vi "Exe_folder_path.vi"(8 "error in (no error)":errorcluster) -> (0 "error out":errorcluster, 2 "One level up":string, 3 "Exe folder":string)   [LabVIEW 2013]
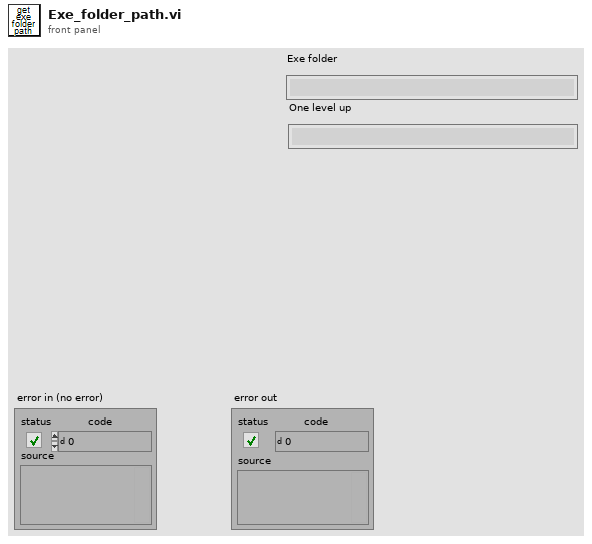
[diagram p1: front panel]
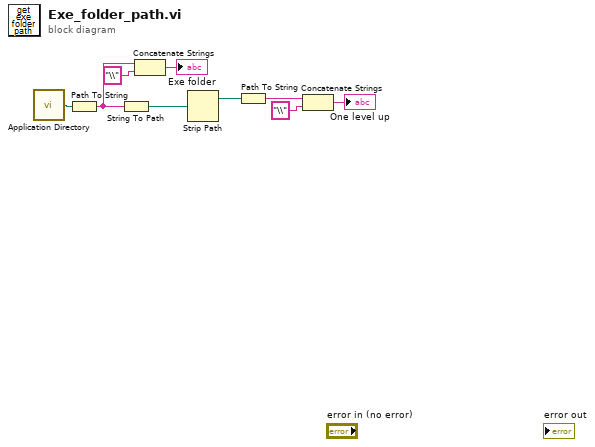
[diagram p0: block diagram]
diagram:
  n1 = call <vilib>:"Application Directory.vi"() -> ("Application Directory"=w9:path)
  n2 = Path To String(path=w9) -> (string=w2:string)
  n3 = String To Path(string=w2) -> (path=w8:path)
  n4 = Concatenate Strings(w2, "\\" ("string")) -> (→"Exe folder":string)
  n5 = Strip Path(path=w8) -> (stripped path=w5:path)  [unwired: 1 out]
  n6 = Path To String(path=w5) -> (string=w7:string)
  n7 = Concatenate Strings(w7, "\\" ("string")) -> (→"One level up":string)
